vi "LogFile.vi"() -> ()   [LabVIEW 2020]
panel:
  out "offset (in records)":i64
  out "record(s)":cluster{"Data 1":string, "Data 2":string}[](array[cluster])
  out "# of records":i64
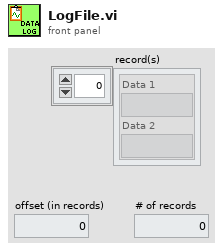
[diagram p1: front panel]
types:
  T1 = enum16{"open", "replace", "create", "open or create", "replace or create", "replace or create with confirmation"}
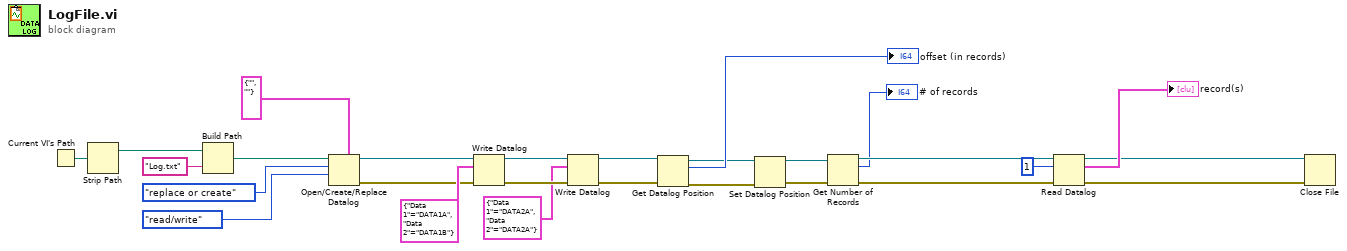
[diagram p0: block diagram]
diagram:
  n1 = Current VI's Path() -> (path=w26:path)
  n2 = Strip Path(path=w26) -> (stripped path=w25:path)  [unwired: 1 out]
  n3 = Build Path(base path=w25, name or relative path="Log.txt") -> (appended path=w23:path)
  n4 = Open/Create/Replace Datalog(5:cluster{"Data 1":string, "Data 2":string} {"Data 1"="", "Data 2"=""} ("Cluster"), 9:enum16{"read/write", "read-only", "write-only"}."read/write" ("access (0:read/write)"), 10:T1."replace or create" ("operation (0:open)"), 11:w23) -> (0:w18:errorcluster, 3:w20:refnum<k1>)  [unwired: 2 in, 1 out]
  n5 = Write Datalog(4:w18, 6:cluster{"Data 1":string, "Data 2":string} {"Data 1"="DATA1A", "Data 2"="DATA1B"} ("record(s)"), 7:w20) -> (0:w17:errorcluster, 3:w16:refnum<k1>)
  n6 = Write Datalog(4:w17, 6:cluster{"Data 1":string, "Data 2":string} {"Data 1"="DATA2A", "Data 2"="DATA2A"} ("record(s)"), 7:w16) -> (0:w8:errorcluster, 3:w9:refnum<k1>)
  n7 = Get Datalog Position(4:w8, 7:w9) -> (0:w6:errorcluster, 2:→"offset (in records)":i64, 3:w5:refnum<k1>)
  n8 = Set Datalog Position(4:w6, 7:w5) -> (0:w3:errorcluster, 3:w4:refnum<k1>)  [unwired: 2 in]
  n9 = Get Number of Records(4:w3, 7:w4) -> (0:w13:errorcluster, 2:→"# of records":i64, 3:w14:refnum<k1>)
  n10 = Read Datalog(4:w13, 6:1 ("count (1)"), 7:w14) -> (0:w2:errorcluster, 2:→"record(s)":cluster{"Data 1":string, "Data 2":string}[], 3:w1:refnum<k1>)
  n11 = Close File(refnum=w1, error in=w2) -> ()  [unwired: 2 out]
